vi "read_digital_worker_loop.vi"(7 "data_queues":T1, 8 "error in (no error)":errorcluster, 9 "data_notifiers":T2, 10 "Notifiers":T4, 11 "Message Queues":T3) -> (0 "error out":errorcluster)   [LabVIEW 2017]
uses:
  support/Notifiers/Notifiers.ctl
  support/Message Queue/All Message Queues.ctl
  support/Message Queue/Message Cluster.ctl
  support/data_notifiers/data_Notifiers.ctl
  measurement_data/MeasurementDatalvclass.lvclass
  support/data_queue/all_data_queue.ctl
  support/measurement_state.ctl
  measurement/Measurement.lvclass
  digital_sim_hardware/DigitalSimHardware.lvclass
  home/minh/Workspace/LDC/Zylinderkopfpruefstand/code/server/hardware/Hardware.lvclass
  hardware/hardware_type.ctl
  support/Message Queue/Enqueue Message (Single).vi
  <vilib>/Utility/error.llb/Error Cluster From Error Code.vi
  <vilib>/ErrorRing/Error Ring.xnode
  support/Message Queue/Message Queue.lvlib
  hardware/Hardware.lvclass
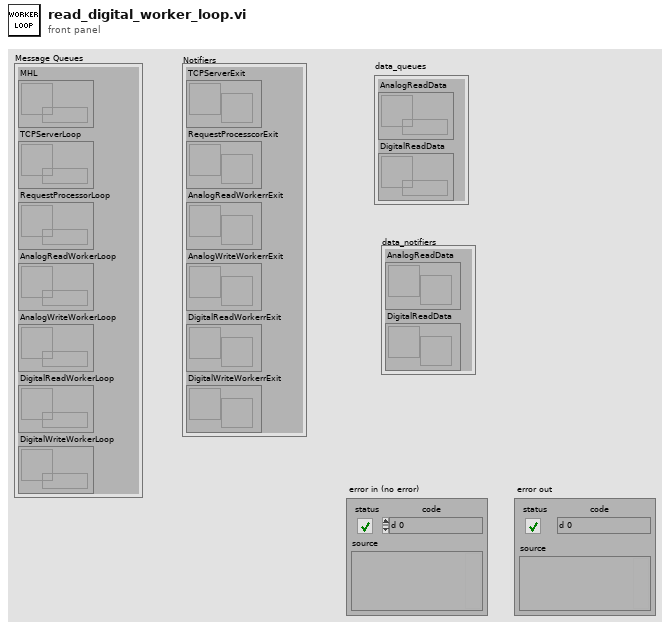
[diagram p1: front panel]
types:
  T1 = typedef "all_data_queue.ctl" = cluster{"AnalogReadData":refnum<queue>, "DigitalReadData":refnum<queue>}
  T2 = typedef "data_Notifiers.ctl" = cluster{"AnalogReadData":refnum<notifier>, "DigitalReadData":refnum<notifier>}
  T3 = typedef "Message Queue.lvlib/All Message Queues.ctl" = cluster{"MHL":refnum<queue>, "TCPServerLoop":refnum<queue>, "RequestProcessorLoop":refnum<queue>, "AnalogReadWorkerLoop":refnum<queue>, "AnalogWriteWorkerLoop":refnum<queue>, "DigitalReadWorkerLoop":refnum<queue>, "DigitalWriteWorkerLoop":refnum<queue>}
  T4 = typedef "Notifiers.ctl" = cluster{"TCPServerExit":refnum<notifier>, "RequestProcesscorExit":refnum<notifier>, "AnalogReadWorkerrExit":refnum<notifier>, "AnalogWriteWorkerrExit":refnum<notifier>, "DigitalReadWorkerrExit":refnum<notifier>, "DigitalWriteWorkerrExit":refnum<notifier>}
  T5 = typedef "measurement_state.ctl" = enum16{"idle", "running"}
  T6 = typedef "Hardware.lvclass/hardware_type.ctl" = enum16{"Analog_Sim_Hardware", "Digital_Sim_Hardware", "AI_Ni_Hardware", "AO_Ni_Hardware", "DI_Ni_Hardware", "DO_Ni_Hardware"}
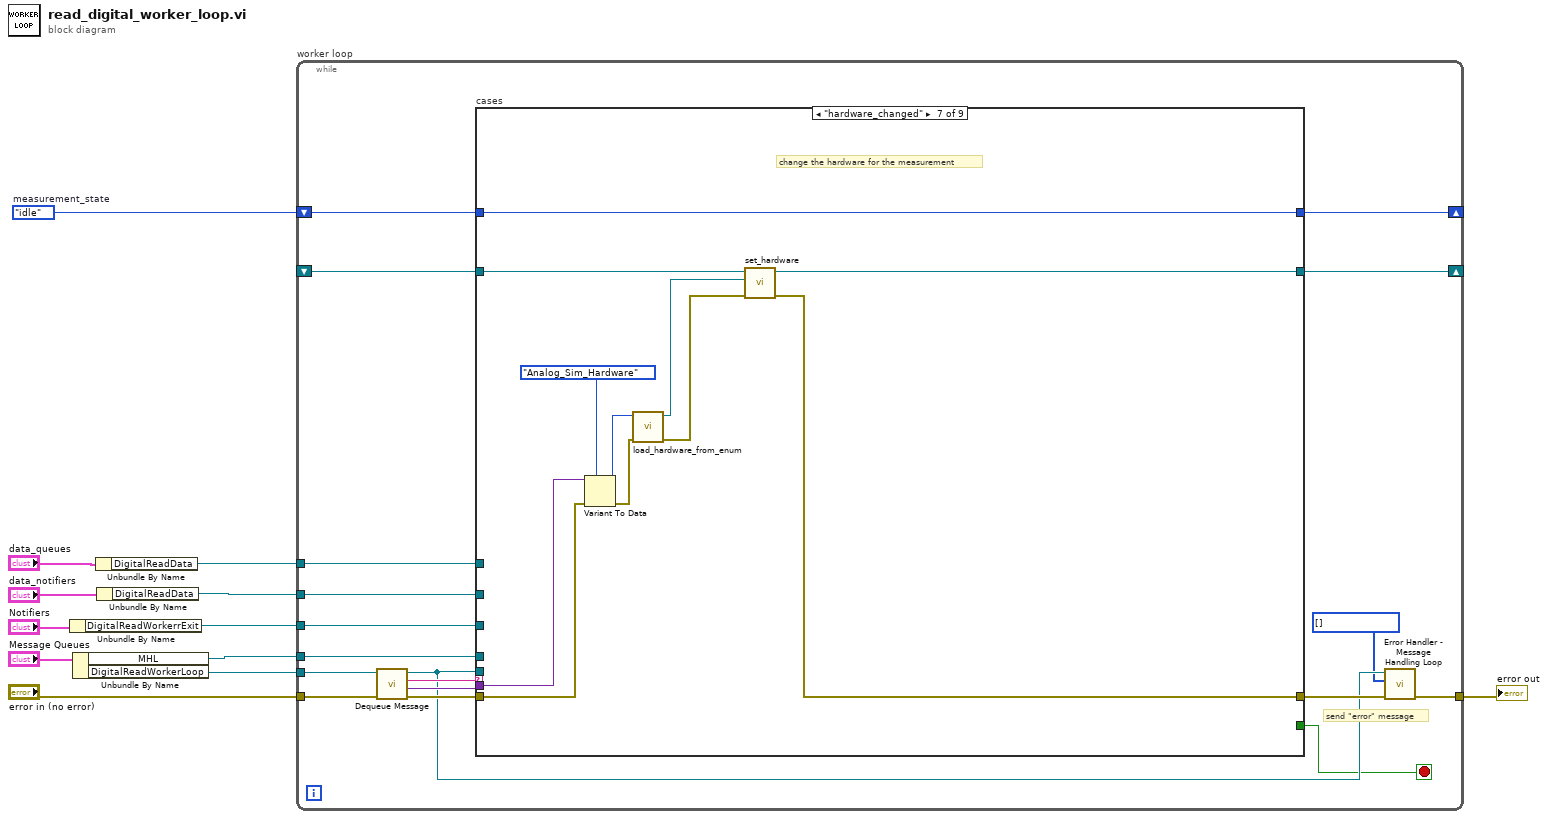
[diagram p0: block diagram]
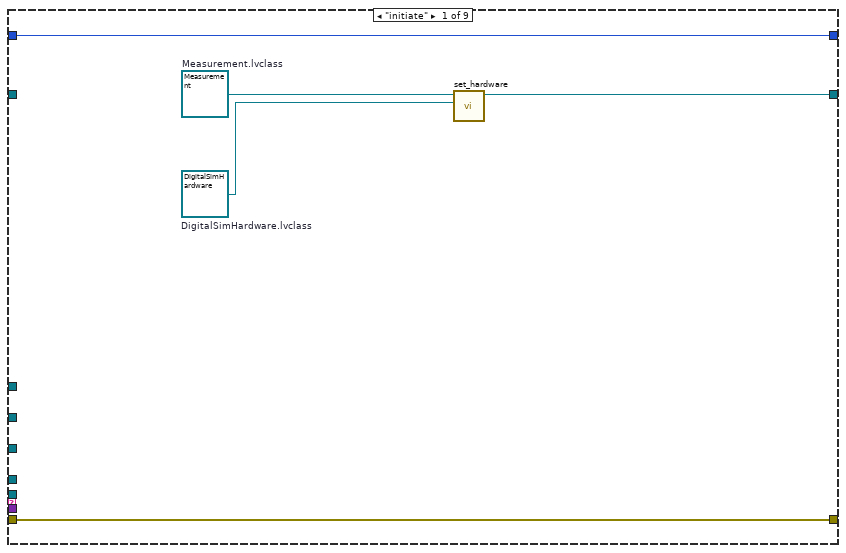
[diagram p2: hidden frame]
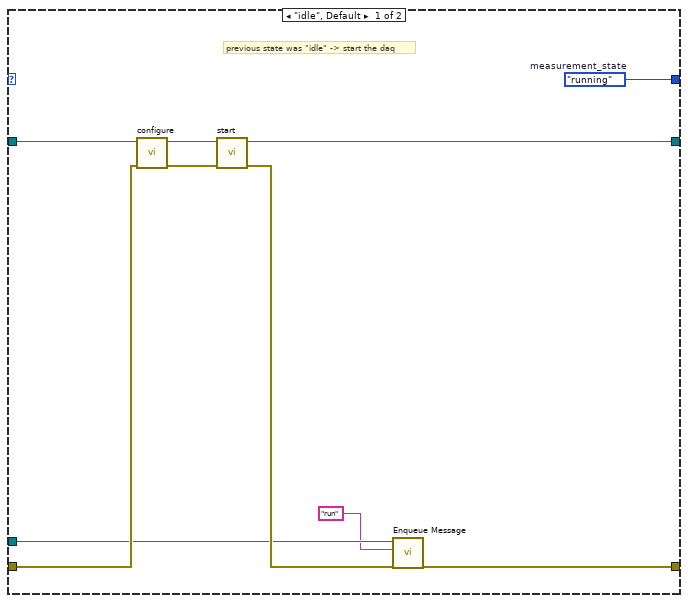
[diagram p4: hidden frame]
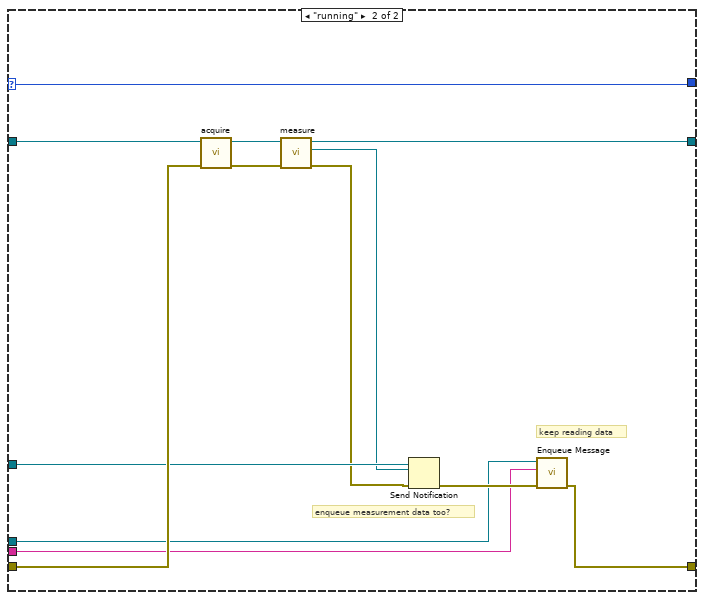
[diagram p6: hidden frame]
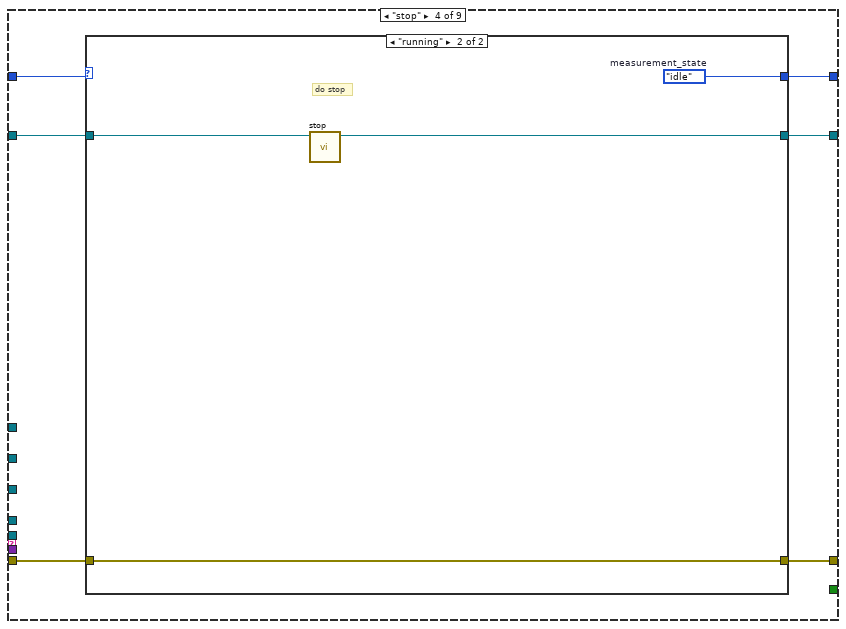
[diagram p7: hidden frame]
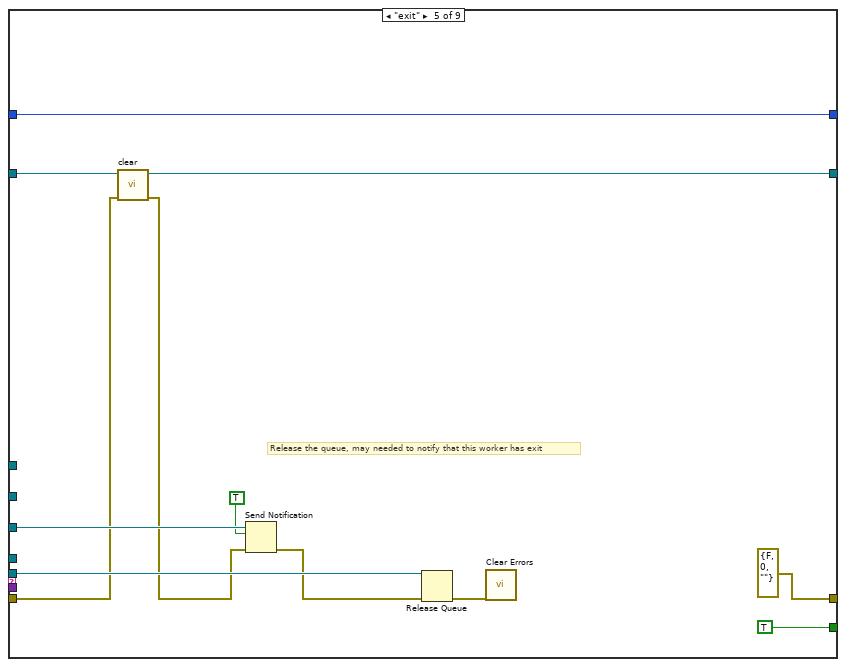
[diagram p9: hidden frame]
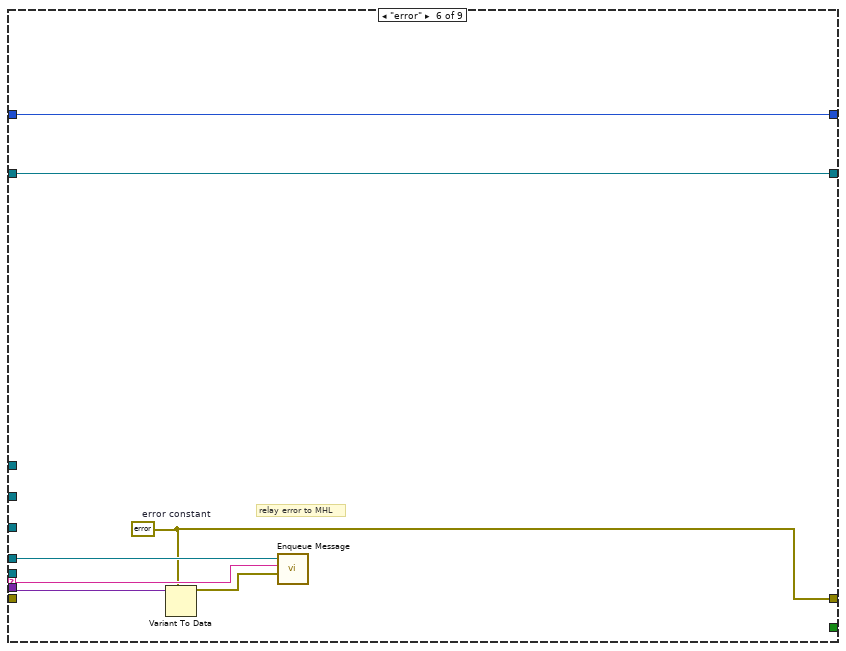
[diagram p10: hidden frame]
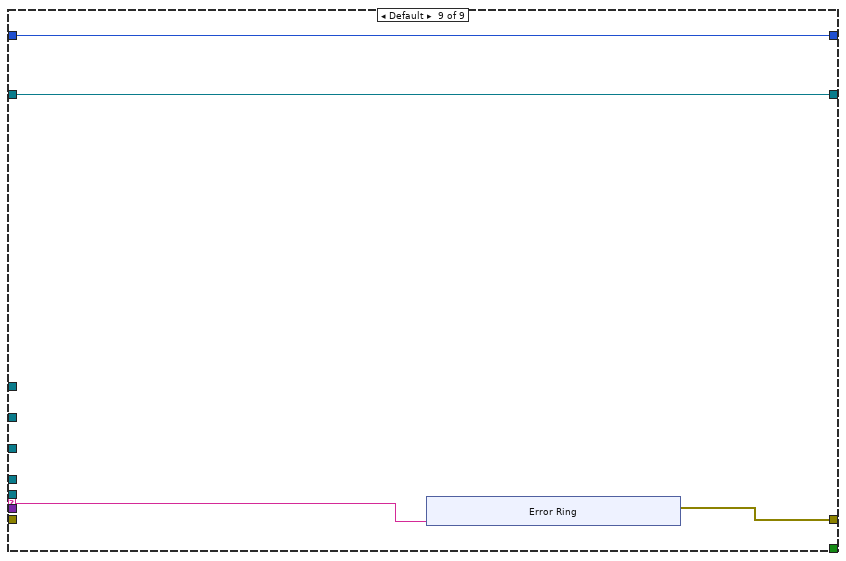
[diagram p12: hidden frame]
diagram:
  w5 = measurement_state."idle"  # measurement_state
  n1 = Unbundle By Name("Notifiers") -> ("DigitalReadWorkerrExit"=w6:refnum<notifier>)
  n2 = Unbundle By Name("Message Queues") -> ("MHL"=w8:refnum<queue>, "DigitalReadWorkerLoop"=w9:refnum<queue>)
  n3 = Unbundle By Name("data_queues") -> ("DigitalReadData"=w2:refnum<queue>)
  n4 = Unbundle By Name("data_notifiers") -> ("DigitalReadData"=w3:refnum<notifier>)
  n5 = while "worker loop" {
    tunnel: "error in (no error)" -> [w30]
    tunnel: [w25] -> w11
    tunnel: w9 -> [w21]
    tunnel: w8 -> [w20]
    tunnel: w6 -> [w19]
    shift-right: [w17] -> _
    shift-left: w5 -> [w18]
    shift-right: [w16] -> _
    shift-left: _ -> [w15]
    tunnel: w3 -> [w14]
    tunnel: w2 -> [w13]
    stop <- w22 stop-if-true
    # "send \"error\" message"
    n6 = call "Dequeue Message.vi"("error in (no error)"=w30, "Message Queue"=w21) -> ("error out"=w29:errorcluster, "Message Data"=w27:variant, "Message"=w28:string, "dup Message Queue"=w24:refnum<queue>)  [unwired: 6 in]
    n7 = case "cases" shown="\"hardware_changed\"" w28 {
      selector: w28 -> [_ _ w56 _ _ w112 _ _ w130]
      tunnel: w29 -> [w35 w42 w62 w86 w96 _ w117 w126 _]
      tunnel: [w35 w41 w61 w85 errorcluster {"status"=FALSE, "code"=0, "source"=""} ("error constant") w108 w120 w126 w129] -> w26
      tunnel: w27 -> [_ _ _ _ _ w111 w118 _ _]
      tunnel: w24 -> [_ w36 w57 _ w103 _ _ _ _]
      tunnel: [_ _ _ _ TRUE _ _ _ _] -> w22
      tunnel: w20 -> [_ _ _ _ _ w109 _ _ _]
      tunnel: w19 -> [_ _ _ _ w102 _ _ _ _]
      tunnel: w18 -> [w34 w40 w64 w84 w99 w107 w123 w125 w128]
      tunnel: [w34 w39 w63 w83 w99 w107 w123 w125 w128] -> w17
      tunnel: [w32 w37 w59 w81 w97 w106 w121 w124 w127] -> w16
      tunnel: w15 -> [_ w38 w60 w82 w98 w106 w122 w124 w127]
      tunnel: w14 -> [_ _ w58 _ _ _ _ _ _]
      tunnel: w13 -> [_ _ _ _ _ _ _ _ _]
      frame "initiate" {
        w31 = refnum<class "DigitalSimHardware.lvclass"> refnum  # DigitalSimHardware.lvclass
        w33 = refnum<class "Measurement.lvclass"> refnum  # Measurement.lvclass
        n8 = call "set_hardware.vi"("new_hardware"=w31, "Measurement in"=w33) -> ("Measurement out"=w32:refnum<class "Measurement.lvclass">)  [unwired: 8 in, 1 out]
      }
      frame "start" {
        n9 = case shown="\"running\"" w40 {
          selector: w40 -> [_ w54]
          tunnel: w42 -> [w48 w55]
          tunnel: [w45 w55] -> w41
          tunnel: [w52 w54] -> w39
          tunnel: w38 -> [w50 w53]
          tunnel: [w51 w53] -> w37
          tunnel: w36 -> [w44 _]
          frame "idle", Default {
            w52 = measurement_state."running"  # measurement_state
            # "previous state was \"idle\" -> start the daq"
            n10 = call-dynamic "configure.vi"("error in (no error)"=w48, "Measurement in"=w50) -> ("error out"=w47:errorcluster, "Measurement out"=w49:refnum<class "Measurement.lvclass">)  [unwired: 8 in]
            n11 = call-dynamic "start.vi"("error in (no error)"=w47, "Measurement in"=w49) -> ("error out"=w46:errorcluster, "Measurement out"=w51:refnum<class "Measurement.lvclass">)  [unwired: 8 in]
            n12 = call-poly "Enqueue Message.vi"("error in (no error)"=w46, "Message"="run", "Message Queue"=w44) -> ("error out"=w45:errorcluster)  [unwired: 7 in, 1 out]
          }
          frame "running" {
            # "already running -> do nothing"
          }
        }
      }
      frame "run" {
        n13 = case shown="\"idle\", Default" w64 {
          selector: w64 -> [w67 w80]
          tunnel: [w67 w80] -> w63
          tunnel: w62 -> [w66 w78]
          tunnel: [w66 w68] -> w61
          tunnel: w60 -> [w65 w79]
          tunnel: [w65 w76] -> w59
          tunnel: w58 -> [_ w74]
          tunnel: w57 -> [_ w70]
          tunnel: w56 -> [_ w69]
          frame "idle", Default {
            # "do nothing"
          }
          frame "running" {
            # "keep reading data"
            # "enqueue measurement data too?"
            n14 = call-dynamic "acquire.vi"("error in (no error)"=w78, "Measurement in"=w79) -> ("error out"=w75:errorcluster, "Measurement out"=w77:refnum<class "Measurement.lvclass">)  [unwired: 8 in]
            n15 = call-dynamic "measure.vi"("error in (no error)"=w75, "Measurement in"=w77) -> ("error out"=w72:errorcluster, "result"=w73:refnum<class "MeasurementDatalvclass.lvclass">, "Measurement out"=w76:refnum<class "Measurement.lvclass">)  [unwired: 7 in]
            n16 = Send Notification(notification=w73, notifier=w74, error in (no error)=w72) -> (error out=w71:errorcluster)  [unwired: 1 out]
            n17 = call-poly "Enqueue Message.vi"("error in (no error)"=w71, "Message"=w69, "Message Queue"=w70) -> ("error out"=w68:errorcluster)  [unwired: 7 in, 1 out]
          }
        }
      }
      frame "stop" {
        n18 = case shown="\"running\"" w84 {
          selector: w84 -> [w88 _]
          tunnel: w86 -> [w89 w93]
          tunnel: [w89 w93] -> w85
          tunnel: [w88 w92] -> w83
          tunnel: w82 -> [w87 w91]
          tunnel: [w87 w90] -> w81
          frame "idle", Default {
            # "do nothing"
          }
          frame "running" {
            w92 = measurement_state."idle"  # measurement_state
            # "do stop"
            n19 = call-dynamic "stop.vi"("Measurement in"=w91) -> ("Measurement out"=w90:refnum<class "Measurement.lvclass">)  [unwired: 9 in, 1 out]
          }
        }
      }
      frame "exit" {
        # "Release the queue, may needed to notify that this worker has exit"
        n20 = call-dynamic "clear.vi"("error in (no error)"=w96, "Measurement in"=w98) -> ("error out"=w95:errorcluster, "Measurement out"=w97:refnum<class "Measurement.lvclass">)  [unwired: 8 in]
        n21 = Send Notification(notification=TRUE, notifier=w102, error in (no error)=w95) -> (error out=w101:errorcluster)  [unwired: 1 out]
        n22 = Release Queue(queue=w103, error in (no error)=w101) -> (error out=w94:errorcluster)  [unwired: 1 in, 2 out]
        n23 = call <vilib>:"Clear Errors.vi"("error in (no error)"=w94) -> ()  [unwired: 5 in, 2 out]
      }
      frame "error" {
        w108 = errorcluster {"status"=FALSE, "code"=0, "source"=""}  # error constant
        # "relay error to MHL"
        n24 = Variant To Data(type=w108, Variant=w111) -> (data=w110:errorcluster)  [unwired: 1 in, 1 out]
        n25 = call-poly "Enqueue Message.vi"("Message Data"=w110, "Message"=w112, "Message Queue"=w109) -> ()  [unwired: 7 in, 2 out]
      }
      frame "hardware_changed" {
        # "change the hardware for the measurement"
        n26 = Variant To Data(error in=w117, type=hardware_type."Analog_Sim_Hardware" ("hardware type"), Variant=w118) -> (data=w116:T6, error out=w114:errorcluster)
        n27 = call "load_hardware_from_enum.vi"("error in (no error)"=w114, "hardware type"=w116) -> ("error out"=w113:errorcluster, "Hardware out"=w115:refnum<class "Hardware.lvclass">)  [unwired: 8 in]
        n28 = call "set_hardware.vi"("error in (no error)"=w113, "new_hardware"=w115, "Measurement in"=w122) -> ("error out"=w120:errorcluster, "Measurement out"=w121:refnum<class "Measurement.lvclass">)  [unwired: 7 in]
      }
      frame "duplicate_me" {
      }
      frame Default {
        n29 = xnode "Error Ring"("parameter 0"=w130) -> ("error out"=w129:errorcluster)
      }
    }
    n30 = call "Error Handler - Message Handling Loop.vi"("error in (no error)"=w26, "Ignore Errors (Runtime)"=i32[] [], "Message Queue"=w24) -> ("dup error in"=w25:errorcluster)  [unwired: 7 in, 1 out]
  }
  "error out" <- w11
